vi "Determine More Warnings.vi"(6 "Max Wind Speed":dbl, 7 "Current Wind Speed":dbl, 9 "Min Temp":dbl, 10 "Max Temp":dbl, 11 "Current Temp":dbl) -> (1 "Warning?":bool, 2 "Warning Text":string)   [LabVIEW 2014]
doc: "This VI is an exercise in the LabVIEW Core I course. In this exercise, you generate appropriate strings for Freeze, Heat Stroke, and High Wind warnings, and combinations of the warnings."
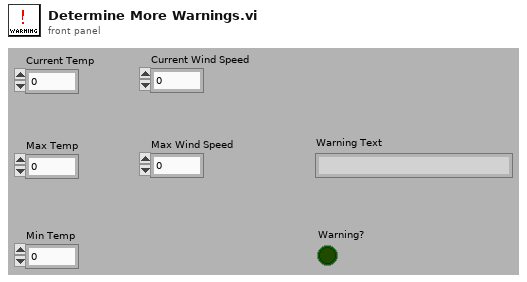
[diagram p1: front panel]
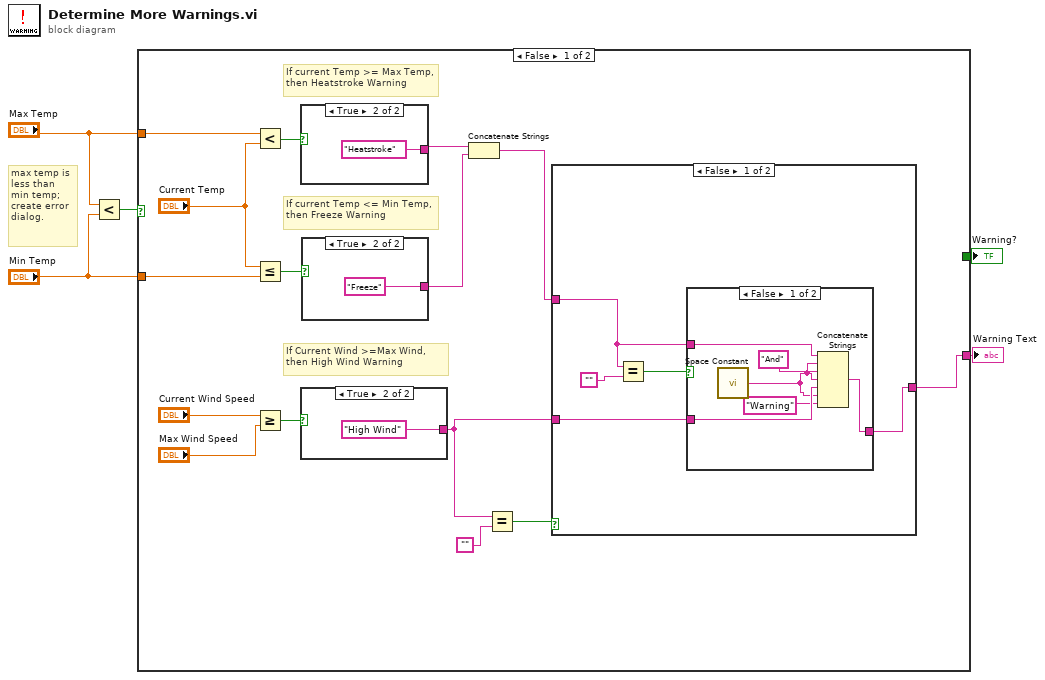
[diagram p0: block diagram]
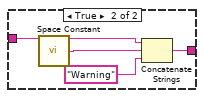
[diagram p2: hidden frame]
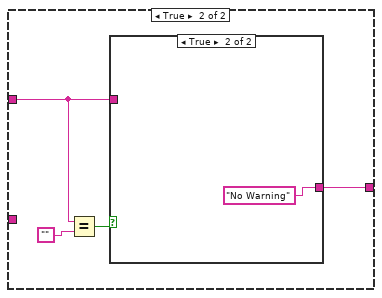
[diagram p3: hidden frame]
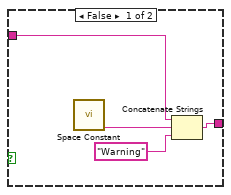
[diagram p4: hidden frame]
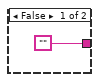
[diagram p5: hidden frame]
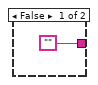
[diagram p6: hidden frame]
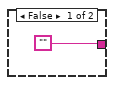
[diagram p7: hidden frame]
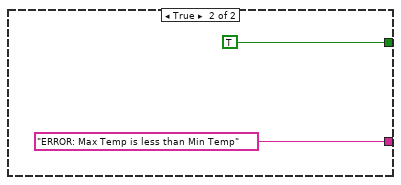
[diagram p8: hidden frame]
diagram:
  # "max temp is less than min temp; create error dialog."
  n1 = Less?(x="Max Temp", y="Min Temp") -> (x < y?=w1:bool)
  n2 = case shown="False" w1 {
    tunnel: [_ TRUE] -> w5
    tunnel: [w10 "ERROR: Max Temp is less than Min Temp"] -> w4
    tunnel: "Max Temp" -> [w14 _]
    tunnel: "Min Temp" -> [w13 _]
    frame False {
      # "If Current Wind >=Max Wind, then High Wind Warning"
      # "If current Temp <= Min Temp, then Freeze Warning"
      # "If current Temp >= Max Temp, then Heatstroke Warning"
      n3 = Less?(x=w14, y="Current Temp") -> (x < y?=w18:bool)
      n4 = Less Or Equal?(x="Current Temp", y=w13) -> (x <= y?=w20:bool)
      n5 = Greater Or Equal?(x="Current Wind Speed", y="Max Wind Speed") -> (x >= y?=w15:bool)
      n6 = case shown="True" w18 {
        tunnel: ["" "Heatstroke"] -> w12
        frame False {
        }
        frame True {
        }
      }
      n7 = case shown="True" w15 {
        tunnel: ["" "High Wind"] -> w6
        frame False {
        }
        frame True {
        }
      }
      n8 = case shown="True" w20 {
        tunnel: ["" "Freeze"] -> w11
        frame False {
        }
        frame True {
        }
      }
      n9 = Concatenate Strings(w12, w11) -> (w9:string)
      n10 = Equal?(x=w6, y="") -> (x = y?=w8:bool)
      n11 = case shown="False" w8 {
        tunnel: [w24 w38] -> w10
        tunnel: w9 -> [w21 w37]
        tunnel: w6 -> [w25 _]
        frame False {
          n12 = Equal?(x=w21, y="") -> (x = y?=w23:bool)
          n13 = case shown="False" w23 {
            tunnel: w25 -> [w29 w33]
            tunnel: [w31 w32] -> w24
            tunnel: w21 -> [w30 _]
            frame False {
              n14 = call <vilib>:"Space Constant.vi"() -> ("String"=w26:string)
              n15 = Concatenate Strings(w30, w26, "And", w26, w29, w26, "Warning") -> (w31:string)
            }
            frame True {
              n16 = call <vilib>:"Space Constant.vi"() -> ("String"=w34:string)
              n17 = Concatenate Strings(w33, w34, "Warning") -> (w32:string)
            }
          }
        }
        frame True {
          n18 = Equal?(x=w37, y="") -> (x = y?=w39:bool)
          n19 = case shown="True" w39 {
            tunnel: [w43 "No Warning"] -> w38
            tunnel: w37 -> [w40 _]
            frame False {
              n20 = call <vilib>:"Space Constant.vi"() -> ("String"=w41:string)
              n21 = Concatenate Strings(w40, w41, "Warning") -> (w43:string)
            }
            frame True {
            }
          }
        }
      }
    }
    frame True {
    }
  }
  "Warning Text" <- w4
  "Warning?" <- w5
